vi "GEOM_ReadDetAmps.vi"(8 "error in (no error)":errorcluster, 9 "detrows":i32, 10 "detcols":i32, 11 "file path":path=path "/home/ArcVIEW/Modules/Geometry/database/TYPES/Hawaii-II_4ch.typ") -> (0 "error out":errorcluster, 2 "amplifiers":T2[](array[typedef]) {"fliped" items=["none", "horizontal", "vertical"]; "type" items=["LL", "LR", "UL", "UR"]}, 3 "cofile path out":path=path "/home/ArcVIEW/Modules/Geometry/database/TYPES/Hawaii-II_4ch.chp", 4 "numxamps":i32, 5 "numyamps":i32)   [LabVIEW 2016]
uses:
  GEOM_Amplifier.ctl
  GEOM_AmpType.ctl
  GEOM_ROI.ctl
  GEOM_Coords.ctl
  <vilib>/Utility/config.llb/Read Key (String).vi
  <vilib>/Utility/config.llb/NI_LVConfig.lvlib
panel:
  in  "type":T1 items=["LL", "LR", "UL", "UR"]
  in  "amplifier":T2={"number"=0, "type"=0, "rotated"=0, "fliped"=0, "FPAcoord"={"xstart"=1, "ystart"=1}, "Physical_size"={"columns"=0, "rows"=0}, "predata"={"columns"=0, "rows"=0}, "postdata"={"columns"=0, "rows"=0}, "Req ROIs"=[], "Corr ROI"=[], "Detnumber"=0, "ampID"="", "discard"=0} {"fliped" items=["none", "horizontal", "vertical"]; "type" items=["LL", "LR", "UL", "UR"]}
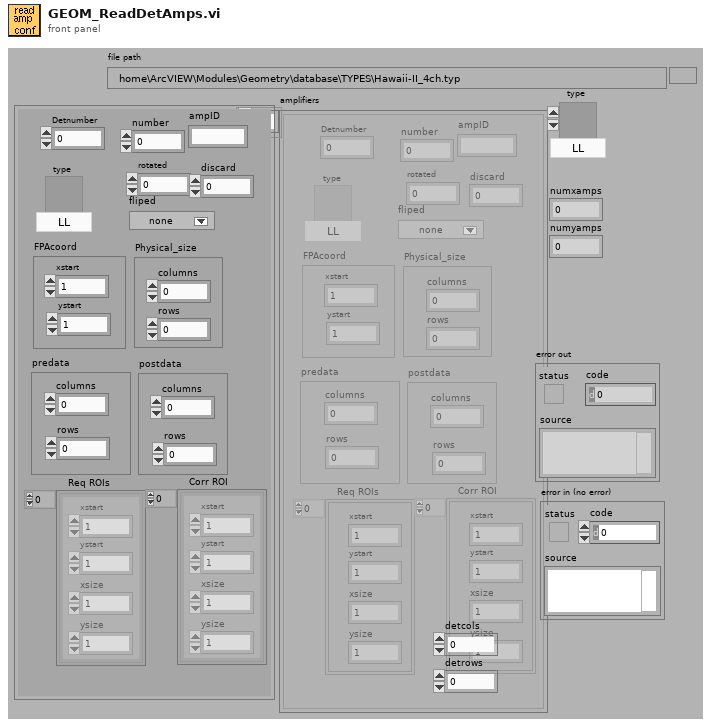
[diagram p1: front panel]
types:
  T1 = typedef "GEOM_AmpType.ctl" = u16
  T2 = typedef "GEOM_Amplifier.ctl" = cluster{"number":i32, "type":T1, "rotated":i16, "fliped":u16, "FPAcoord":cluster{"xstart":i32, "ystart":i32}, "Physical_size":cluster{"columns":i32, "rows":i32}, "predata":cluster{"columns":i32, "rows":i32}, "postdata":cluster{"columns":i32, "rows":i32}, "Req ROIs":T3, "Corr ROI":T3, "Detnumber":i32, "ampID":string, "discard":i32}
  T3 = typedef "GEOM_ROI.ctl" = T4[]
  T4 = typedef "GEOM_Coords.ctl" = cluster{"xstart":u32, "ystart":u32, "xsize":u32, "ysize":u32}
  T5 = typedef "NI_LVConfig.lvlib/Config Data RefNum.ctl" = refnum<k1>
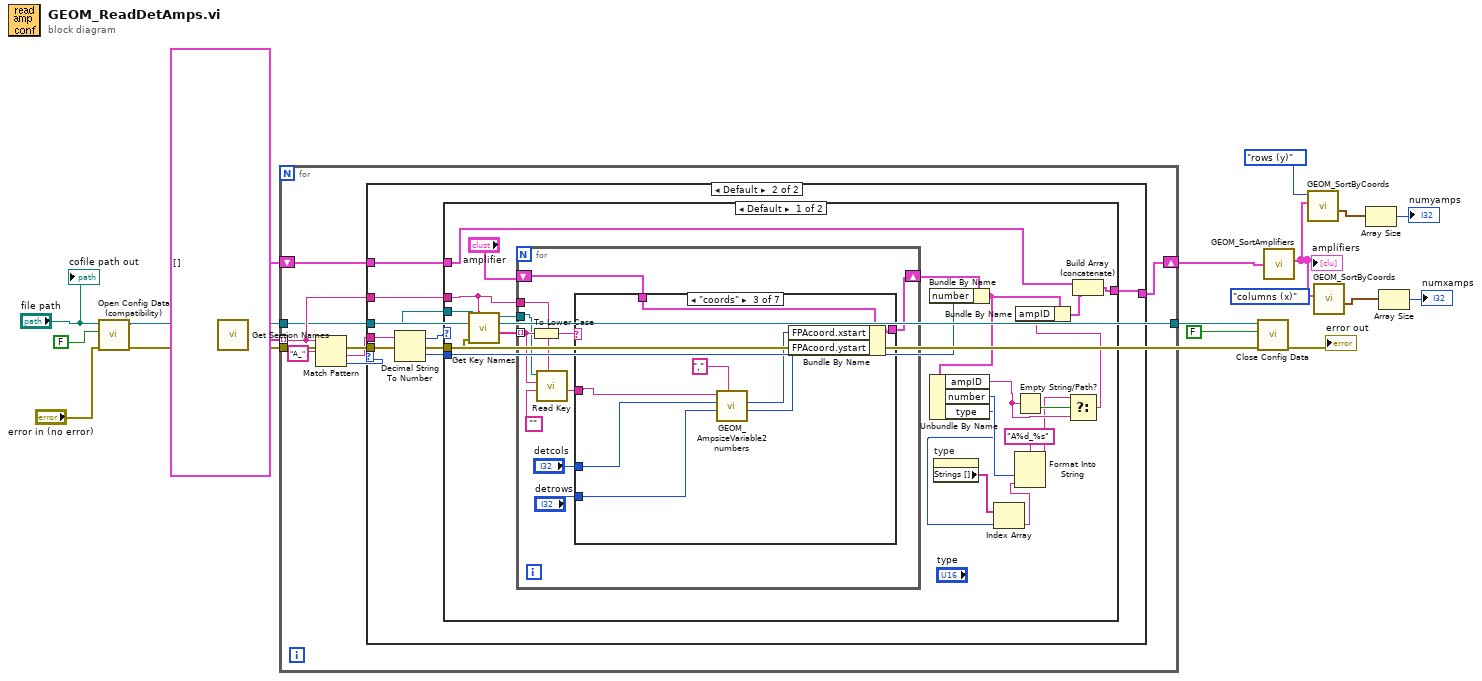
[diagram p0: block diagram]
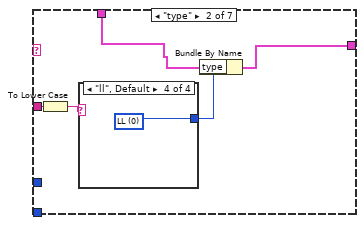
[diagram p4: hidden frame]
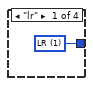
[diagram p5: hidden frame]
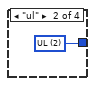
[diagram p6: hidden frame]
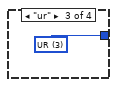
[diagram p7: hidden frame]
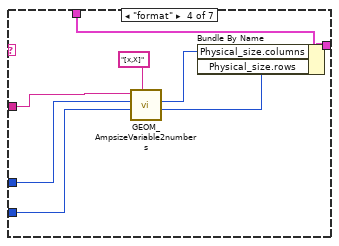
[diagram p8: hidden frame]
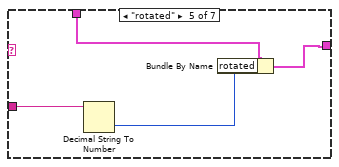
[diagram p9: hidden frame]
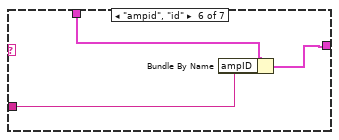
[diagram p10: hidden frame]
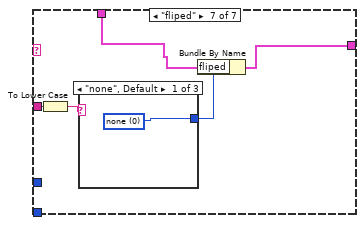
[diagram p11: hidden frame]
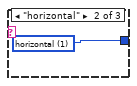
[diagram p12: hidden frame]
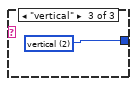
[diagram p13: hidden frame]
diagram:
  n1 = call <vilib>:"Open Config Data (compatibility).vi"("error in (no error)"="error in (no error)", "create file if necessary (T)"=FALSE ("create file if necessary? (T)"), "configuration file path"="file path") -> ("error out"=w16:errorcluster, "refnum"=w17:T5)  [unwired: 6 in, 1 out]
  n2 = call <vilib>:"Get Section Names.vi"("error in (no error)"=w16, "refnum"=w17) -> ("error out"=w13:errorcluster, "section names"=w18:string[], "refnum out"=w19:T5)  [unwired: 7 out]
  n3 = for {
    tunnel: w19 -> [w22]
    tunnel: w18 -> [w25] mode=indexing
    shift-right: [w24] -> w11
    shift-left: T2[] [] -> [w23]
    tunnel: [w22] -> w15
    tunnel: w13 -> [w21]
    n4 = Match Pattern(string=w25, regular expression="A_") -> (after substring=w26:string, offset past match=w27:i32)  [unwired: 3 out]
    n5 = case shown="Default" w27 {
      tunnel: w26 -> [_ w37]
      tunnel: w25 -> [_ w35]
      tunnel: w22 -> [_ w34]
      tunnel: [w29 w31] -> w24
      tunnel: w23 -> [w29 w32]
      tunnel: w21 -> [_ w30]
      frame -1 {
      }
      frame Default {
        n6 = Decimal String To Number(string=w37) -> (offset past number=w36:i32, number=w33:i32)  [unwired: 2 out]
        n7 = case shown="Default" w36 {
          tunnel: w35 -> [w56 _]
          tunnel: w34 -> [w58 _]
          tunnel: w33 -> [w47 _]
          tunnel: w32 -> [w50 w110]
          tunnel: [w53 w110] -> w31
          tunnel: w30 -> [w51 _]
          frame Default {
            n8 = call <vilib>:"Get Key Names.vi"("section"=w56, "error in (no error)"=w51, "refnum"=w58) -> ("key names"=w57:string[], "refnum out"=w52:T5)  [unwired: 7 out]
            n9 = for {
              tunnel: w57 -> [w66] mode=indexing
              tunnel: w56 -> [w67]
              shift-right: [w62] -> w54
              shift-left: "amplifier" -> [w63]
              tunnel: w52 -> [w61]
              n10 = To Lower Case(string=w66) -> (all lower case string=w68:string)
              n11 = call-poly <vilib>:"Read Key.vi"("section"=w67, "default value"="", "key"=w66, "refnum"=w61) -> ("value"=w64:string)  [unwired: 2 in, 5 out]
              n12 = case shown="\"coords\"" w68 {
                tunnel: w64 -> [_ w73 w84 w92 w96 w99 w105]
                tunnel: w63 -> [w69 w74 w86 w94 w98 w101 w106]
                tunnel: [w69 w70 w85 w93 w97 w100 w102] -> w62
                tunnel: "detcols" -> [_ _ w80 w90 _ _ _]
                tunnel: "detrows" -> [_ _ w79 w89 _ _ _]
                frame Default {
                }
                frame "type" {
                  n13 = To Lower Case(string=w73) -> (all lower case string=w72:string)
                  n14 = case shown="\"ll\", Default" w72 {
                    tunnel: [w75 w76 w77 w78] -> w71
                    frame "lr" {
                      w75 = u16 1 items=["LL", "LR", "UL", "UR"] ("type")
                    }
                    frame "ul" {
                      w76 = u16 2 items=["LL", "LR", "UL", "UR"] ("type")
                    }
                    frame "ur" {
                      w77 = u16 3 items=["LL", "LR", "UL", "UR"] ("type")
                    }
                    frame "ll", Default {
                      w78 = u16 0 items=["LL", "LR", "UL", "UR"] ("type")
                    }
                  }
                  n15 = Bundle By Name(cluster=w74, "type"=w71) -> (w70:T2)
                }
                frame "coords" {
                  n16 = call "GEOM_AmpsizeVariable2numbers.vi"("separator"=",", "detrows"=w79, "detcols"=w80, "ampval"=w84) -> ("amprows"=w81:i32, "ampcols"=w82:i32)  [unwired: 6 out]
                  n17 = Bundle By Name(cluster=w86, "FPAcoord.xstart"=w82, "FPAcoord.ystart"=w81) -> (w85:T2)
                }
                frame "format" {
                  n18 = call "GEOM_AmpsizeVariable2numbers.vi"("separator"="[x,X]" ("regular expression"), "detrows"=w89, "detcols"=w90, "ampval"=w92) -> ("amprows"=w87:i32, "ampcols"=w88:i32)  [unwired: 6 out]
                  n19 = Bundle By Name(cluster=w94, "Physical_size.columns"=w88, "Physical_size.rows"=w87) -> (w93:T2)
                }
                frame "rotated" {
                  n20 = Decimal String To Number(string=w96) -> (number=w95:i32)  [unwired: 3 out]
                  n21 = Bundle By Name(cluster=w98, "rotated"=w95) -> (w97:T2)
                }
                frame "ampid", "id" {
                  n22 = Bundle By Name(cluster=w101, "ampID"=w99) -> (w100:T2)
                }
                frame "fliped" {
                  n23 = To Lower Case(string=w105) -> (all lower case string=w104:string)
                  n24 = case shown="\"none\", Default" w104 {
                    tunnel: [w107 w108 w109] -> w103
                    frame "none", Default {
                      w107 = u16 0 items=["none", "horizontal", "vertical"] ("fliped")
                    }
                    frame "horizontal" {
                      w108 = u16 1 items=["none", "horizontal", "vertical"] ("fliped")
                    }
                    frame "vertical" {
                      w109 = u16 2 items=["none", "horizontal", "vertical"] ("fliped")
                    }
                  }
                  n25 = Bundle By Name(cluster=w106, "fliped"=w103) -> (w102:T2)
                }
              }
            }
            n26 = Bundle By Name(cluster=w54, "number"=w47) -> (w46:T2)
            n27 = Unbundle By Name(w46) -> ("ampID"=w48:string, "number"=w41:i32, "type"=w39:T1)
            n28 = property on="type" class="Ring (strict)"() -> ("Strings []"=w40:string[])  [unwired: 2 in, 2 out]
            n29 = Index Array(array=w40, index=w39) -> (element=w38:string)
            n30 = Empty String/Path?(string/path=w48) -> (empty?=w49:bool)
            n31 = Format Into String(format string="A%d_%s", w41, w38) -> (resulting string=w43:string)  [unwired: 2 in, 1 out]
            n32 = Select(t=w43, s=w49, f=w48) -> (s? t:f=w44:string)
            n33 = Bundle By Name(cluster=w46, "ampID"=w44) -> (w45:T2)
            n34 = Build Array (concatenate)(w50, w45) -> (w53:T2[])
          }
          frame -1 {
          }
        }
      }
    }
  }
  n35 = call <vilib>:"Close Config Data.vi"("error in (no error)"=w13, "write file if changed (T)"=FALSE ("write configuration file? (T)"), "refnum"=w15) -> ("error out"=→"error out":errorcluster)  [unwired: 8 out]
  n36 = call "GEOM_SortAmplifiers.vi"("amplifiers"=w11) -> ("sorted amplifiers"=w6:T2[])  [unwired: 10 out]
  "amplifiers" <- w6
  n37 = call "GEOM_SortByCoords.vi"("amplifiers"=w6, "how"=enum16{"rows (y)", "columns (x)"}."rows (y)") -> ("levels"=w2:cluster{"amplifiers":i32, "coord":i32}[])  [unwired: 9 out]
  n38 = call "GEOM_SortByCoords.vi"("amplifiers"=w6, "how"=enum16{"rows (y)", "columns (x)"}."columns (x)") -> ("levels"=w4:cluster{"amplifiers":i32, "coord":i32}[])  [unwired: 9 out]
  n39 = Array Size(array=w2) -> (size(s)=→"numyamps":i32)
  n40 = Array Size(array=w4) -> (size(s)=→"numxamps":i32)
  "cofile path out" <- "file path"
